vi "EnFlo_Tunnel_Global.vi"() -> ()   [LabVIEW 2018]
panel:
  in  "Minimum Ref Velocity for taking Results":dbl=0.4
  in  "Minimum Shaft RPM":dbl=30.0
  in  "Minimum Ref Velocity":dbl=0.004
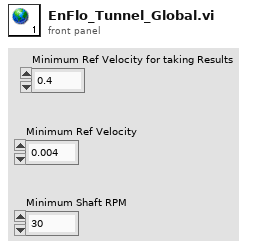
[diagram p1: front panel]
diagram:
